vi "toml_value_uint.vi"(5 "operation":T1, 6 "modifiers":u16 format="%016b", 7 "section":string[](array[string]), 8 "error in (no error)":errorcluster, 9 "value in":u64, 10 "key":string[](array[string]), 11 "path in":path) -> (0 "error out":errorcluster, 1 "value out":u64, 2 "exists?":bool, 3 "path out":path)   [LabVIEW 2017]
uses:
  toml_value_operation.ctl
  toml_fg_action.ctl
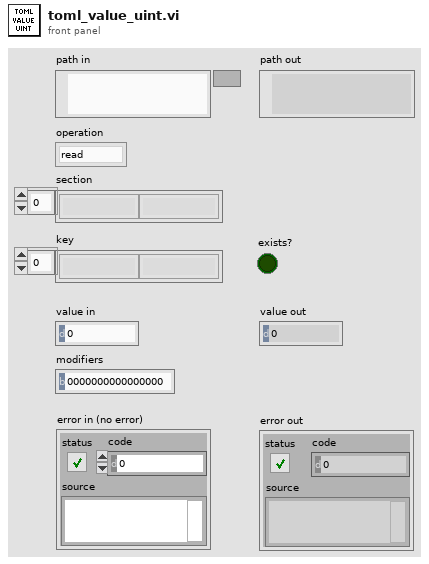
[diagram p1: front panel]
types:
  T1 = typedef "toml_value_operation.ctl" = enum8{"read", "write", "delete"}
  T2 = typedef "toml_fg_action.ctl" = enum8{"null", "get", "set", "pop", "import", "export", "drop"}
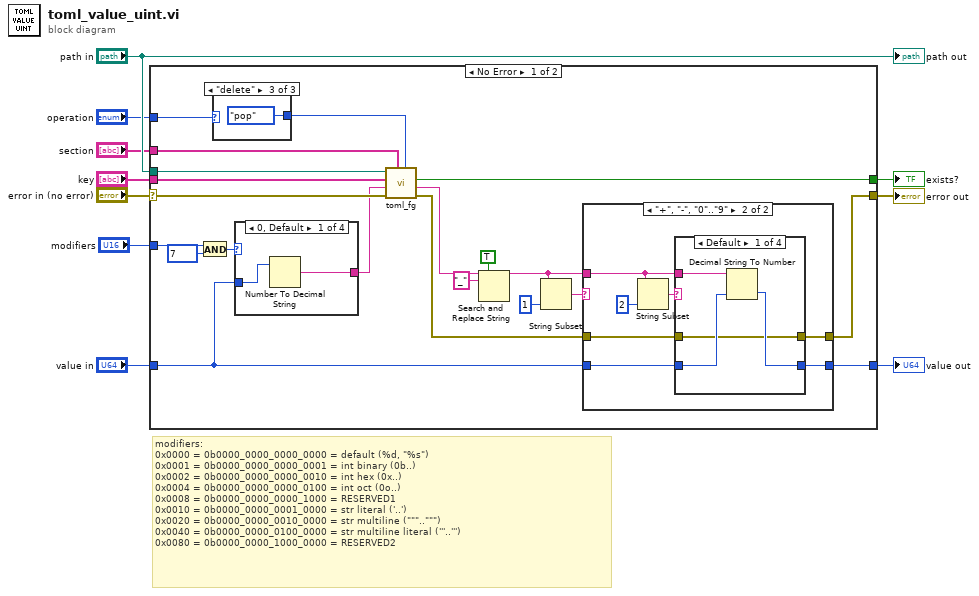
[diagram p0: block diagram]
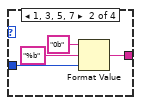
[diagram p2: hidden frame]
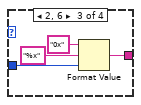
[diagram p3: hidden frame]
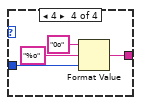
[diagram p4: hidden frame]
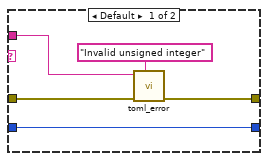
[diagram p5: hidden frame]
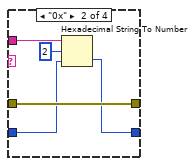
[diagram p6: hidden frame]
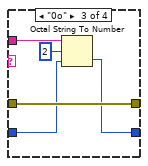
[diagram p7: hidden frame]
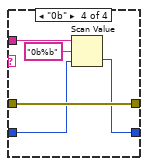
[diagram p8: hidden frame]
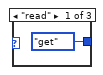
[diagram p9: hidden frame]
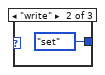
[diagram p10: hidden frame]
diagram:
  # "modifiers:\n0x0000 = 0b0000_0000_0000_0000 = default (%d, \"%s\")\n0x0001 = 0b0000_0000_0000_0001 = int binary (0b..)\n0x0002 = 0b0000_0000_0000_0010 = int hex (0x..)\n0x0004 = 0b0000_0000_0000_0100 = int oct (0o..)\n0x0008 = 0b0000_0000_0000_1000 = RESERVED1\n0x0010 = 0b0000_0000_0001_0000 = str literal ('..')\n0x0020 = 0b0000_0000_0010_0000 = str multiline (\"\"\"..\"\"\")\n0x0040 = 0b0000_0000_0100_0000 = str multiline literal ('''..''')\n0x0080 = 0b0000_0000_1000_0000 = RESERVED2"
  n1 = case shown="No Error" "error in (no error)" {
    selector: "error in (no error)" -> [w31 w81]
    tunnel: [w22 w81] -> w9
    tunnel: "path in" -> [w30 _]
    tunnel: "operation" -> [w28 _]
    tunnel: "section" -> [w27 _]
    tunnel: "key" -> [w26 _]
    tunnel: [w25 _] -> w4
    tunnel: [w24 w80] -> w3
    tunnel: "value in" -> [w21 w80]
    tunnel: "modifiers" -> [w17 _]
    frame No Error {
      n2 = And(x=w17, y=u16 7) -> (x .and. y?=w16:u16)
      n3 = case shown="\"delete\"" w28 {
        tunnel: [toml_fg_action."get" ("action") toml_fg_action."set" ("action") toml_fg_action."pop" ("action")] -> w29
        frame "read" {
        }
        frame "write" {
        }
        frame "delete" {
        }
      }
      n4 = case shown="0, Default" w16 {
        tunnel: w21 -> [w33 w36 w40 w44]
        tunnel: [w32 w37 w41 w45] -> w20
        frame 0, Default {
          n5 = Number To Decimal String(number=w33) -> (decimal integer string=w32:string)  [unwired: 1 in]
        }
        frame 1, 3, 5, 7 {
          n6 = Format Value(string ("")="0b", format string="%b", value (0)=w36) -> (output string=w37:string)
        }
        frame 2, 6 {
          n7 = Format Value(string ("")="0x", format string="%x", value (0)=w40) -> (output string=w41:string)
        }
        frame 4 {
          n8 = Format Value(string ("")="0o", format string="%o", value (0)=w44) -> (output string=w45:string)
        }
      }
      n9 = call "toml_fg.vi"("action"=w29, "section"=w27, "error in (no error)"=w31, "value in"=w20, "key"=w26, "path in"=w30) -> ("error out"=w23:errorcluster, "value out"=w14:string, "exists?"=w25:bool)  [unwired: 2 in, 1 out]
      n10 = Search and Replace String(replace all?=TRUE ("replace all? (F)"), input string=w14, search string="_") -> (result string=w13:string)  [unwired: 5 in, 3 out]
      n11 = String Subset(string=w13, length (rest)=1 ("length (rest)")) -> (substring=w18:string)  [unwired: 1 in]
      n12 = case shown="\"+\", \"-\", \"0\"..\"9\"" w18 {
        tunnel: [w47 w51] -> w24
        tunnel: [w49 w56] -> w22
        tunnel: w23 -> [w50 w55]
        tunnel: w21 -> [w47 w52]
        tunnel: w13 -> [w46 w53]
        frame Default {
          n13 = call "toml_error.vi"("message"="Invalid unsigned integer", "error in (no error)"=w50, "toml"=w46) -> ("error out"=w49:errorcluster)  [unwired: 8 in]
        }
        frame "+", "-", "0".."9" {
          n14 = String Subset(string=w53, length (rest)=2 ("length (rest)")) -> (substring=w54:string)  [unwired: 1 in]
          n15 = case shown="Default" w54 {
            tunnel: [w58 w66 w71 w76] -> w56
            tunnel: w55 -> [w58 w66 w71 w76]
            tunnel: w53 -> [w61 w65 w70 w75]
            tunnel: w52 -> [w60 w64 w69 w74]
            tunnel: [w59 w63 w68 w73] -> w51
            frame Default {
              n16 = Decimal String To Number(string=w61, default (0L)=w60) -> (number=w59:u64)  [unwired: 1 in, 1 out]
            }
            frame "0x" {
              n17 = Hexadecimal String To Number(string=w65, offset=2, default (0uL)=w64) -> (number=w63:u64)  [unwired: 1 out]
            }
            frame "0o" {
              n18 = Octal String To Number(2:w69, 3:2 ("offset"), 4:w70) -> (0:w68:u64)  [unwired: 1 out]
            }
            frame "0b" {
              n19 = Scan Value(string=w75, format string="0b%b", default (0 dbl)=w74) -> (value=w73:u64)  [unwired: 1 out]
            }
          }
        }
      }
    }
    frame Error {
    }
  }
  "error out" <- w9
  "value out" <- w3
  "exists?" <- w4
  "path out" <- "path in"
